vi "Calculate_Mean.vi"(8 "error in":errorcluster) -> (0 "error out":errorcluster, 2 "Mean":dbl format="%0.6f")   [LabVIEW 2020]
uses:
  <vilib>/Analysis/baseanly.llb/Mean (DBL).vi
  <vilib>/Analysis/NI_AALBase.lvlib
panel:
  out "Array":dbl[](array[numeric])
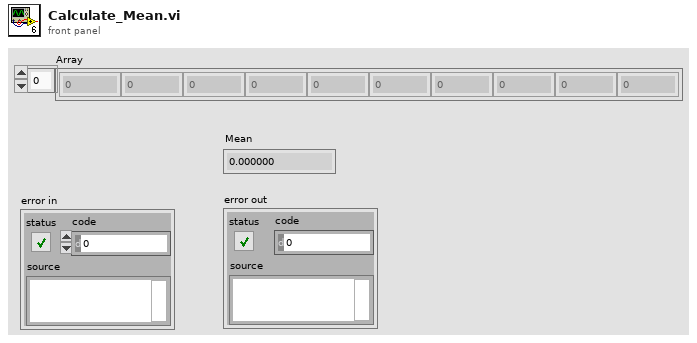
[diagram p1: front panel]
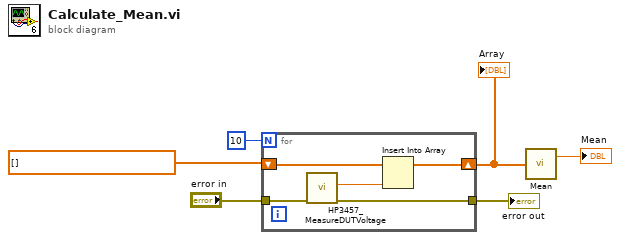
[diagram p0: block diagram]
diagram:
  n1 = for {
    N: 10 -> [_]
    shift-right: [w11] -> w5
    shift-left: dbl[] [] -> [w10]
    tunnel: "error in" -> [w8]
    tunnel: [w7] -> w2
    n2 = call "HP3457_MeasureDUTVoltage.vi"("error in"=w8) -> ("error out"=w7:errorcluster, "DUTVoltage"=w9:dbl)  [unwired: 8 in]
    n3 = Insert Into Array(array=w10, new element=w9) -> (w11:dbl[])  [unwired: 1 in]
  }
  "error out" <- w2
  "Array" <- w5
  n4 = call-poly <vilib>:"Mean.vi"("X"=w5) -> ("mean"=→"Mean":dbl)  [unwired: 1 out]
